vi "get overlapping banking transaction.vi"(8 "error in (no error)":errorcluster, 10 "Importing Transactions":refnum<class "Statement.lvclass">, 11 "Database in":refnum<class "Database.lvclass">) -> (0 "error out":errorcluster, 2 "Overlapping Records":refnum<class "Statement.lvclass">, 3 "Database out":refnum<class "Database.lvclass">)   [LabVIEW 2018, in "Database.lvclass"]
uses:
  Database.lvclass
  Statement/Statement.lvclass
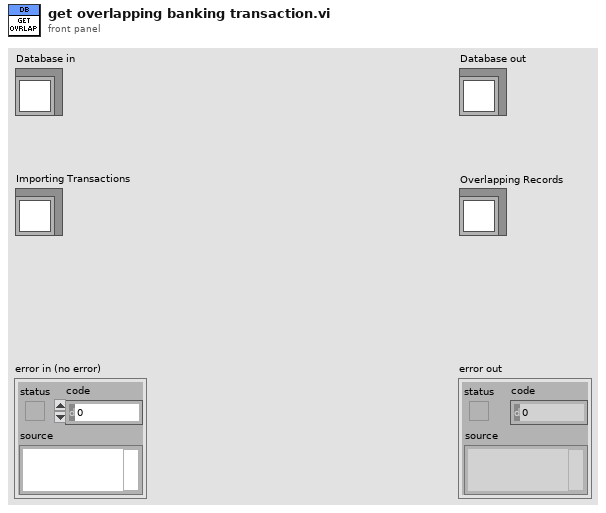
[diagram p1: front panel]
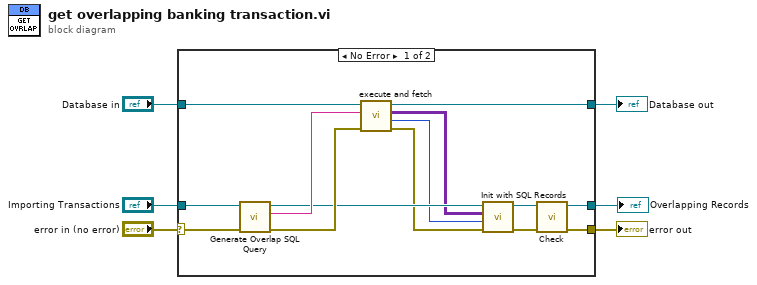
[diagram p0: block diagram]
diagram:
  n1 = case shown="No Error" "error in (no error)" {
    selector: "error in (no error)" -> [w18 w22]
    tunnel: [w7 w22] -> w5
    tunnel: [w19 w21] -> w3
    tunnel: "Database in" -> [w20 w21]
    tunnel: [w8 _] -> w2
    tunnel: "Importing Transactions" -> [w14 _]
    frame No Error {
      n2 = call-dynamic "Generate Overlap SQL Query.vi"("error in (no error)"=w18, "Importing Transactions"=w14) -> ("error out"=w17:errorcluster, "Overlap Query"=w16:string, "Overlapping Records"=w15:refnum<class "Statement.lvclass">)  [unwired: 7 in]
      n3 = call "execute and fetch.vi"("error in (no error)"=w17, "SQL query"=w16, "Database in"=w20) -> ("error out"=w13:errorcluster, "Num records"=w11:i32, "recordset data"=w12:variant[][], "Database out"=w19:refnum<class "Database.lvclass">)  [unwired: 5 in]
      n4 = call-dynamic "Init with SQL Records.vi"("error in (no error)"=w13, "Num records"=w11, "SQL Dataset"=w12, "Statement in"=w15) -> ("error out"=w9:errorcluster, "Statement out"=w10:refnum<class "Statement.lvclass">)  [unwired: 6 in]
      n5 = call-dynamic "Check.vi"("error in (no error)"=w9, "Statement in"=w10) -> ("error out"=w7:errorcluster, "Statement out"=w8:refnum<class "Statement.lvclass">)  [unwired: 8 in]
    }
    frame Error {
    }
  }
  "error out" <- w5
  "Database out" <- w3
  "Overlapping Records" <- w2
